vi "hydrolysis_reactor_setup.vi"(10 "#":i32) -> (2 "spec_file":path)   [LabVIEW 2019]
uses:
  lib/libSimulationControl/libSimulationControl.lvlib
  lib/libCheckpointUpdate/libCheckpointUpdate.lvlib
  lib/libFileFunctions/libFileFunctions.lvlib
panel:
  out "inflow path":path
  # "*******************************************************************\nBiogas Plant Control\n\nAuthor: Paul Zügel\nGCSC-Frankfurt am Main 2020\n\n*******************************************************************"
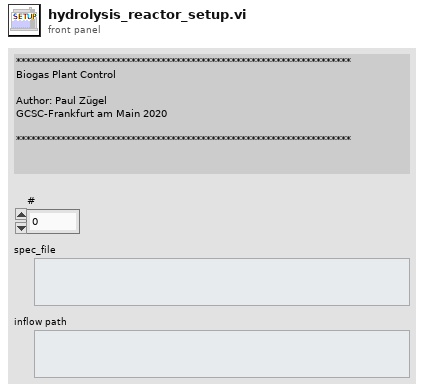
[diagram p1: front panel]
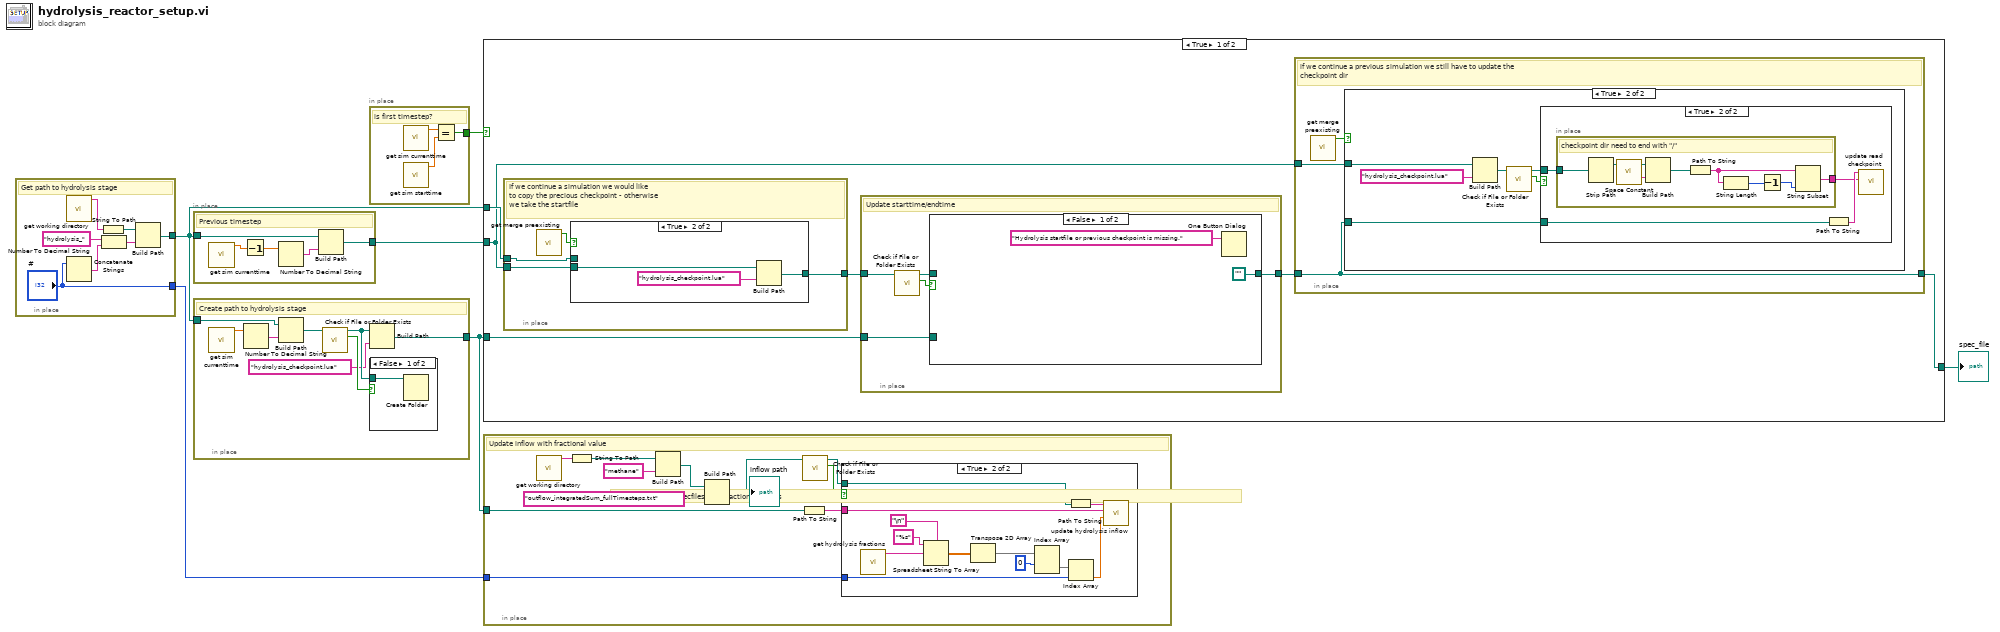
[diagram p0: block diagram]
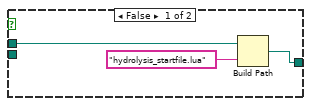
[diagram p4: hidden frame]
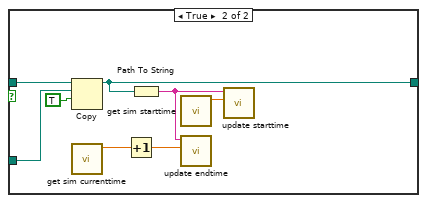
[diagram p5: hidden frame]
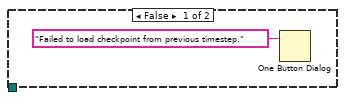
[diagram p7: hidden frame]
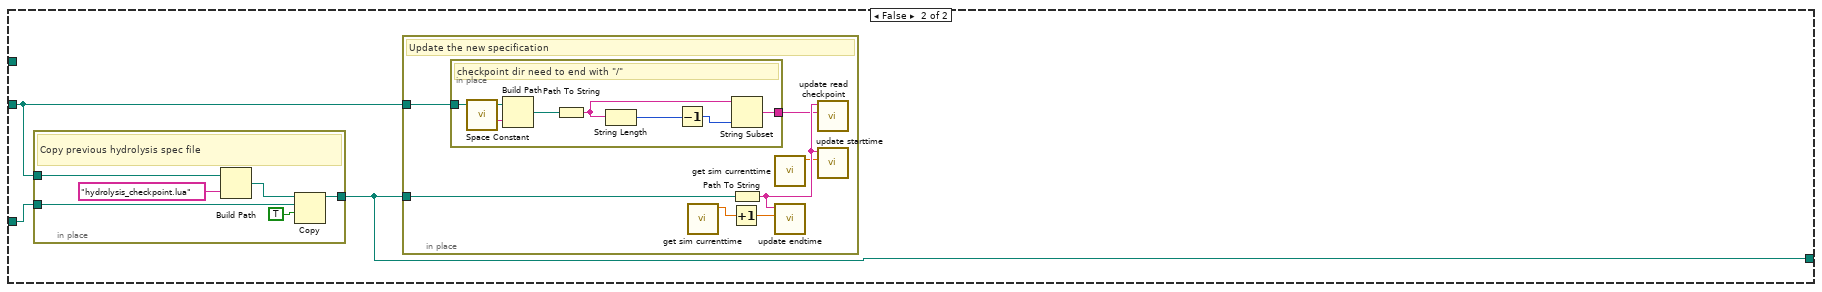
[diagram p8: hidden frame]
diagram:
  n1 = in-place {
    in-place-border: [w8] -> w2
    in-place-border: ["#"] -> w1
    # "Get path to hydrolysis stage"
    n2 = call "get working directory.vi"() -> ("function return"=w12:string)  [unwired: 10 in, 1 out]
    n3 = Number To Decimal String(number="#") -> (decimal integer string=w13:string)  [unwired: 1 in]
    n4 = String To Path(string=w12) -> (path=w9:path)
    n5 = Concatenate Strings("hydrolysis_" ("string"), w13) -> (w11:string)
    n6 = Build Path(base path=w9, name or relative path=w11) -> (appended path=w8:path)
  }
  n7 = in-place {
    in-place-border: [w16] -> w3
    in-place-border: w2 -> [w14]
    # "Previous timestep"
    n8 = call "get sim currenttime.vi"() -> ("current_time"=w15:dbl)  [unwired: 10 in, 1 out]
    n9 = Decrement(x=w15) -> (x-1=w18:dbl)
    n10 = Number To Decimal String(number=w18) -> (decimal integer string=w17:string)  [unwired: 1 in]
    n11 = Build Path(base path=w14, name or relative path=w17) -> (appended path=w16:path)
  }
  n12 = in-place {
    in-place-border: [w21] -> w5
    in-place-border: w2 -> [w19]
    # "Create path to hydrolysis stage"
    n13 = call "get sim currenttime.vi"() -> ("current_time"=w20:dbl)  [unwired: 10 in, 1 out]
    n14 = Number To Decimal String(number=w20) -> (decimal integer string=w25:string)  [unwired: 1 in]
    n15 = Build Path(base path=w19, name or relative path=w25) -> (appended path=w24:path)
    n16 = call <vilib>:"Check if File or Folder Exists.vi"("path"=w24) -> ("file or folder exists?"=w26:bool, "dup path"=w23:path)  [unwired: 8 in, 1 out]
    n17 = Build Path(base path=w23, name or relative path="hydrolysis_checkpoint.lua" ("string")) -> (appended path=w21:path)
    n18 = case shown="False" w26 {
      tunnel: w23 -> [w27 _]
      frame False {
        n19 = Create Folder(path (use dialog)=w27) -> ()  [unwired: 2 in, 3 out]
      }
      frame True {
      }
    }
  }
  n20 = in-place {
    in-place-border: [w30] -> w6
    # "is first timestep?"
    n21 = call "get sim currenttime.vi"() -> ("current_time"=w28:dbl)  [unwired: 10 in, 1 out]
    n22 = call "get sim starttime.vi"() -> ("sim_starttime"=w29:dbl)  [unwired: 10 in, 1 out]
    n23 = Equal?(x=w28, y=w29) -> (x = y?=w30:bool)
  }
  n24 = case shown="True" w6 {
    tunnel: w5 -> [w32 w84]
    tunnel: [w36 w86] -> w4
    tunnel: w3 -> [w33 w85]
    tunnel: w2 -> [w34 _]
    frame True {
      n25 = in-place {
        in-place-border: [w40] -> w35
        in-place-border: w34 -> [w38]
        in-place-border: w33 -> [w37]
        # "If we continue a simulation we would like\nto copy the precious checkpoint - otherwise\nwe take the startfile"
        n26 = call "get merge preexisting.vi"() -> ("function return"=w39:bool)  [unwired: 10 in, 1 out]
        n27 = case shown="True" w39 {
          tunnel: [w42 w45] -> w40
          tunnel: w38 -> [w41 _]
          tunnel: w37 -> [_ w44]
          frame False {
            # "Copy base specification and update starttime/endtime"
            n28 = Build Path(base path=w41, name or relative path="hydrolysis_startfile.lua") -> (appended path=w42:path)
          }
          frame True {
            # "Copy previous hydrolysis spec file"
            n29 = Build Path(base path=w44, name or relative path="hydrolysis_checkpoint.lua" ("string")) -> (appended path=w45:path)
          }
        }
      }
      n30 = in-place {
        in-place-border: w35 -> [w49]
        in-place-border: w32 -> [w48]
        in-place-border: [w47] -> w31
        # "Update starttime/endtime"
        n31 = call <vilib>:"Check if File or Folder Exists.vi"("path"=w49) -> ("file or folder exists?"=w50:bool, "dup path"=w51:path)  [unwired: 8 in, 1 out]
        n32 = case shown="False" w50 {
          tunnel: [path "" w61] -> w47
          tunnel: w51 -> [_ w58]
          tunnel: w48 -> [_ w57]
          frame False {
            n33 = One Button Dialog(message="Hydrolysis startfile or previous checkpoint is missing.") -> ()  [unwired: 1 in, 1 out]
          }
          frame True {
            # "Update starttime/endtime"
            n34 = Copy(9:TRUE ("overwrite (F)"), 10:w57, 11:w58) -> (3:w61:path)  [unwired: 2 in, 2 out]
            n35 = call "get sim currenttime.vi"() -> ("current_time"=w56:dbl)  [unwired: 10 in, 1 out]
            n36 = Increment(x=w56) -> (x+1=w55:dbl)
            n37 = Path To String(path=w61) -> (string=w59:string)
            n38 = call "get sim starttime.vi"() -> ("sim_starttime"=w54:dbl)  [unwired: 10 in, 1 out]
            n39 = call "update endtime.vi"("endtime"=w55, "spec_dir"=w59) -> ()  [unwired: 9 in, 1 out]
            n40 = call "update starttime.vi"("starttime"=w54, "spec_dir"=w59) -> ()  [unwired: 9 in, 1 out]
          }
        }
      }
      n41 = in-place {
        in-place-border: [w62] -> w36
        in-place-border: w33 -> [w63]
        in-place-border: w31 -> [w62]
        # "if we continue a previous simulation we still have to update the \ncheckpoint dir"
        n42 = call "get merge preexisting.vi"() -> ("function return"=w64:bool)  [unwired: 10 in, 1 out]
        n43 = case shown="True" w64 {
          tunnel: w63 -> [_ w69]
          tunnel: w62 -> [_ w65]
          frame False {
          }
          frame True {
            n44 = Build Path(base path=w69, name or relative path="hydrolysis_checkpoint.lua" ("string")) -> (appended path=w68:path)
            n45 = call <vilib>:"Check if File or Folder Exists.vi"("path"=w68) -> ("file or folder exists?"=w66:bool, "dup path"=w67:path)  [unwired: 8 in, 1 out]
            n46 = case shown="True" w66 {
              tunnel: w67 -> [_ w73]
              tunnel: w65 -> [_ w74]
              frame False {
                n47 = One Button Dialog(message="Failed to load checkpoint from previous timestep.") -> ()  [unwired: 1 in, 1 out]
              }
              frame True {
                n48 = in-place {
                  in-place-border: w73 -> [w83]
                  in-place-border: [w76] -> w72
                  # "checkpoint dir need to end with \"/\""
                  n49 = Strip Path(path=w83) -> (stripped path=w77:path)  [unwired: 1 out]
                  n50 = call <vilib>:"Space Constant.vi"() -> ("String"=w78:string)
                  n51 = Build Path(base path=w77, name or relative path=w78) -> (appended path=w81:path)
                  n52 = Path To String(path=w81) -> (string=w82:string)
                  n53 = String Length(string=w82) -> (length=w80:i32)
                  n54 = Decrement(x=w80) -> (x-1=w79:i32)
                  n55 = String Subset(string=w82, length (rest)=w79) -> (substring=w76:string)  [unwired: 1 in]
                }
                n56 = Path To String(path=w74) -> (string=w75:string)
                n57 = call "update read checkpoint.vi"("checkpoint_dir"=w72, "spec_dir"=w75) -> ()  [unwired: 9 in, 1 out]
              }
            }
          }
        }
      }
    }
    frame False {
      n58 = in-place {
        in-place-border: w84 -> [w103]
        in-place-border: [w102] -> w86
        in-place-border: w85 -> [w101]
        # "Copy previous hydrolysis spec file"
        n59 = Build Path(base path=w101, name or relative path="hydrolysis_checkpoint.lua" ("string")) -> (appended path=w105:path)
        n60 = Copy(9:TRUE ("overwrite (F)"), 10:w103, 11:w105) -> (3:w102:path)  [unwired: 2 in, 2 out]
      }
      n61 = in-place {
        in-place-border: w85 -> [w87]
        in-place-border: w86 -> [w89]
        # "Update the new specification"
        n62 = in-place {
          in-place-border: [w95] -> w88
          in-place-border: w87 -> [w94]
          # "checkpoint dir need to end with \"/\""
          n63 = call <vilib>:"Space Constant.vi"() -> ("String"=w96:string)
          n64 = Build Path(base path=w94, name or relative path=w96) -> (appended path=w99:path)
          n65 = Path To String(path=w99) -> (string=w100:string)
          n66 = String Length(string=w100) -> (length=w98:i32)
          n67 = Decrement(x=w98) -> (x-1=w97:i32)
          n68 = String Subset(string=w100, length (rest)=w97) -> (substring=w95:string)  [unwired: 1 in]
        }
        n69 = call "get sim currenttime.vi"() -> ("current_time"=w91:dbl)  [unwired: 10 in, 1 out]
        n70 = Increment(x=w91) -> (x+1=w90:dbl)
        n71 = Path To String(path=w89) -> (string=w93:string)
        n72 = call "get sim currenttime.vi"() -> ("current_time"=w92:dbl)  [unwired: 10 in, 1 out]
        n73 = call "update endtime.vi"("endtime"=w90, "spec_dir"=w93) -> ()  [unwired: 9 in, 1 out]
        n74 = call "update read checkpoint.vi"("checkpoint_dir"=w88, "spec_dir"=w93) -> ()  [unwired: 9 in, 1 out]
        n75 = call "update starttime.vi"("starttime"=w92, "spec_dir"=w93) -> ()  [unwired: 9 in, 1 out]
      }
    }
  }
  "spec_file" <- w4
  n76 = in-place {
    in-place-border: w5 -> [w109]
    in-place-border: w1 -> [w107]
    # "Update inflow with fractional value"
    # "Update hydrolysis specfiles with fractional inflows"
    n77 = call "get working directory.vi"() -> ("function return"=w117:string)  [unwired: 10 in, 1 out]
    n78 = String To Path(string=w117) -> (path=w116:path)
    n79 = Build Path(base path=w116, name or relative path="methane") -> (appended path=w114:path)
    n80 = Build Path(base path=w114, name or relative path="outflow_integratedSum_fullTimesteps.txt") -> (appended path=w112:path)
    "inflow path" <- w112
    n81 = Path To String(path=w109) -> (string=w108:string)
    n82 = call <vilib>:"Check if File or Folder Exists.vi"("path"=w112) -> ("file or folder exists?"=w111:bool, "dup path"=w110:path)  [unwired: 8 in, 1 out]
    n83 = case shown="True" w111 {
      tunnel: w110 -> [_ w129]
      tunnel: w108 -> [_ w128]
      tunnel: w107 -> [_ w119]
      frame False {
      }
      frame True {
        n84 = call "get hydrolysis fractions.vi"() -> ("function return"=w126:string)  [unwired: 10 in, 1 out]
        n85 = Spreadsheet String To Array(delimiter (Tab)="\n", format string="%s", spreadsheet string=w126) -> (array=w124:dbl[][])  [unwired: 1 in]
        n86 = Transpose 2D Array(2D array=w124) -> (transposed array=w125:dbl[][])
        n87 = Index Array(array=w125, index (row)=0) -> (element=w120:dbl[])  [unwired: 1 in]
        n88 = Path To String(path=w129) -> (string=w127:string)
        n89 = Index Array(array=w120, index=w119) -> (element=w118:dbl)
        n90 = call "update hydrolysis inflow.vi"("fraction"=w118, "hydrolysis_specfiles"=w128, "outflow_infile"=w127) -> ()  [unwired: 8 in, 1 out]
      }
    }
  }
